vi "CheckMasterConnection.vi"(3 "Master IP":string="192.168.0.101:11311") -> (0 "error out":errorcluster, 1 "Master There?":bool)   [LabVIEW 2013]
doc: "Returns true if it was able to open a connection to the ROS Master"
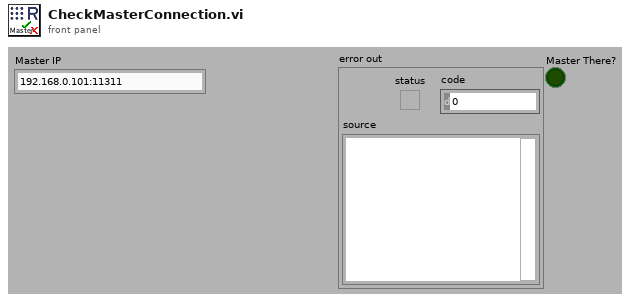
[diagram p1: front panel]
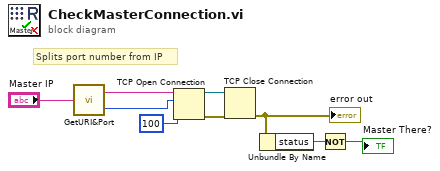
[diagram p0: block diagram]
diagram:
  # "Splits port number from IP"
  n1 = call "GetURI&Port.vi"("URI in"="Master IP") -> ("Port"=w7:u16, "URI"=w8:string)
  n2 = TCP Open Connection(address=w8, remote port or service name=w7, timeout ms (60000)=100) -> (connection ID=w5:refnum<k5>, error out=w6:errorcluster)  [unwired: 2 in]
  n3 = TCP Close Connection(connection ID=w5, error in (no error)=w6) -> (error out=w3:errorcluster)  [unwired: 1 in, 1 out]
  "error out" <- w3
  n4 = Unbundle By Name(w3) -> ("status"=w2:bool)
  n5 = Not(x=w2) -> (.not. x?=→"Master There?":bool)
